vi "Stop Core.vi"(10 "final error code":i32, 11 "Class Loader in":refnum<class "Class Loader.lvclass">) -> (3 "Class Loader out":refnum<class "Class Loader.lvclass">)   [LabVIEW 2023, in "Class Loader.lvlib" / "Class Loader.lvclass"]
doc: "(<B>Filename</B>: Actor Framework.lvlib:Actor.lvclass:Stop Core.vi)\n\nDefines what the actor does before it stops. Use the <B>final error code</B> input to determine whether the actor shut down in response to an error.\n\nBy default, this method passes the Stop message along to all auto-stop nested actors. A descendant class may override this method to define additional behavior, such as shutting down any processes the actor initiated in its override of the Actor Core method."
uses:
  Class Loader.lvclass
  Class Loader.lvclass/Class Loader.ctl
  <userlib>/_OpenG.lib/error/error.llb/openg_error.lvlib
  <vilib>/LS Instruments AG/Async Methods Actor/Async Methods Actor/Async Methods Actor/Async Methods Actor.lvclass
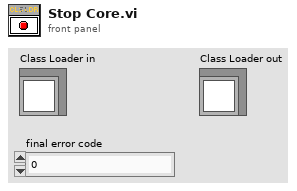
[diagram p1: front panel]
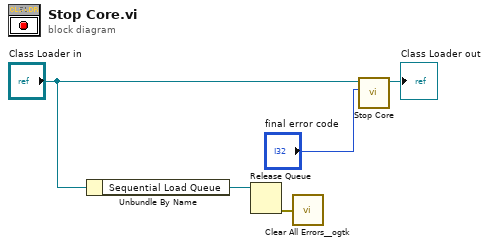
[diagram p0: block diagram]
diagram:
  n1 = Unbundle By Name("Class Loader in") -> ("Sequential Load Queue"=w3:refnum<queue>)
  n2 = Release Queue(queue=w3) -> (error out=w2:errorcluster)  [unwired: 2 in, 2 out]
  n3 = call <userlib>:"Clear All Errors__ogtk.vi"("Error In"=w2) -> ()  [unwired: 3 in, 1 out]
  n4 = call-parent "Stop Core.vi"("final error code"="final error code", "Async Methods Actor in"="Class Loader in") -> ("Async Methods Actor out"=→"Class Loader out":refnum<class "Class Loader.lvclass">)  [unwired: 9 in]
